vi "Obtain Message Queue - Config.vi"(8 "error in (no error)":errorcluster) -> (0 "error out":errorcluster, 3 "Config":refnum<queue>)   [LabVIEW 2017, in "Message Queue.lvlib"]
doc: "Create a queue with the Message Cluster data type."
uses:
  Message Queue.lvlib
  Configuration/Controls/Config Commands.ctl
  Configuration/Controls/ConfigStates.ctl
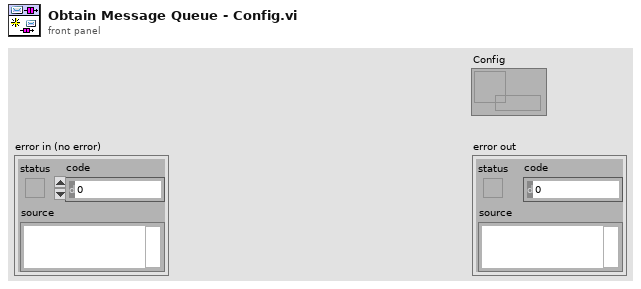
[diagram p1: front panel]
types:
  T1 = typedef "Config Commands.ctl" = cluster{"ConfigStates":T2, "Variant":variant}
  T2 = typedef "ConfigStates.ctl" = enum16{"Init", "Read", "Write"}
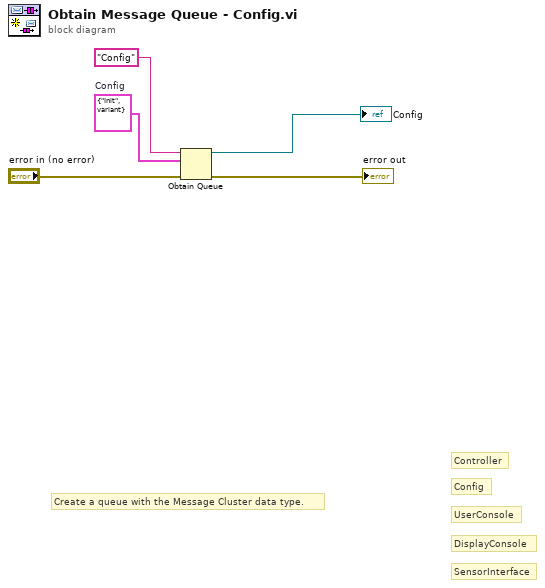
[diagram p0: block diagram]
diagram:
  w3 = T1 {"ConfigStates"=enum."Init", "Variant"=variant}  # Config
  # "SensorInterface"
  # "DisplayConsole"
  # "UserConsole"
  # "Config"
  # "Controller"
  # "Create a queue with the Message Cluster data type."
  n1 = Obtain Queue(name (unnamed)="Config", element data type=w3, error in (no error)="error in (no error)") -> (queue out=→"Config":refnum<queue>, error out=→"error out":errorcluster)  [unwired: 2 in, 1 out]
